vi "Stop Door Actuators.vi"(8 "error in (no error)":errorcluster, 11 "Door Hardware in":refnum<class "Door Hardware.lvclass">) -> (0 "error out":errorcluster, 3 "Door Hardware out":refnum<class "Door Hardware.lvclass">)   [LabVIEW 2020, in "Door Hardware.lvlib" / "Door Hardware.lvclass"]
uses:
  Door Hardware.lvclass
  Door Hardware.lvclass/Door Hardware.ctl
  Door Actuator/Door Actuator.lvclass
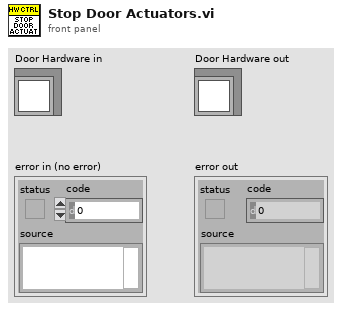
[diagram p1: front panel]
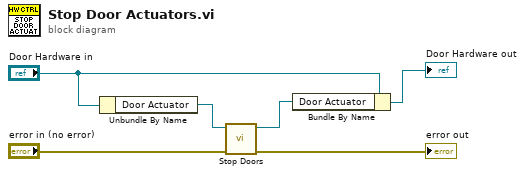
[diagram p0: block diagram]
diagram:
  n1 = Unbundle By Name("Door Hardware in") -> ("Door Actuator"=w6:refnum<class "Door Actuator.lvclass">)
  n2 = call-dynamic "Stop Doors.vi"("error in (no error)"="error in (no error)", "Door Actuator in"=w6) -> ("error out"=→"error out":errorcluster, "Door Actuator out"=w2:refnum<class "Door Actuator.lvclass">)  [unwired: 8 in]
  n3 = Bundle By Name(cluster="Door Hardware in", "Door Actuator"=w2) -> (→"Door Hardware out":refnum<class "Door Hardware.lvclass">)
